vi "Calculate Q0 continous.vi"(8 "error in (no error)":errorcluster, 9 "dt":dbl=1e-06 format="%#_13g", 10 "Data":dbl[][](array[numeric]), 11 "Scope5761 in":refnum<class "Scope5782_six_channel.lvclass">) -> (0 "error out":errorcluster, 1 "Q0 error":bool, 2 "Data out":dbl[][](array[numeric]), 3 "Scope5761out":refnum<class "Scope5782_six_channel.lvclass">)   [LabVIEW 2025, in "Scope5782_six_channel.lvclass"]
uses:
  Scope5782_six_channel.lvclass
  Scope5782_six_channel.lvclass/Scope5782_six_channel.ctl
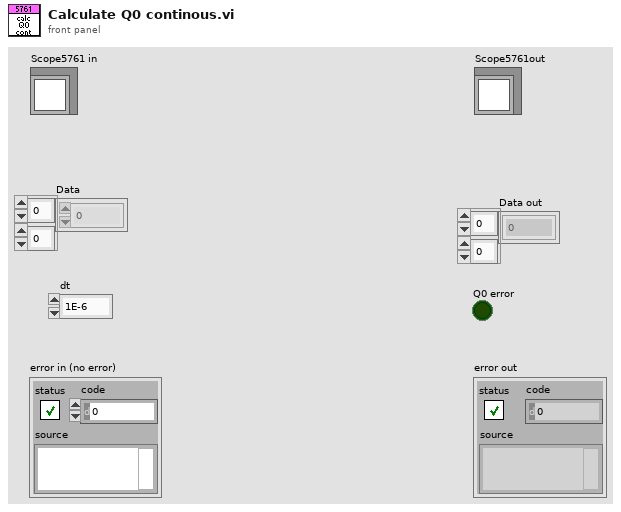
[diagram p1: front panel]
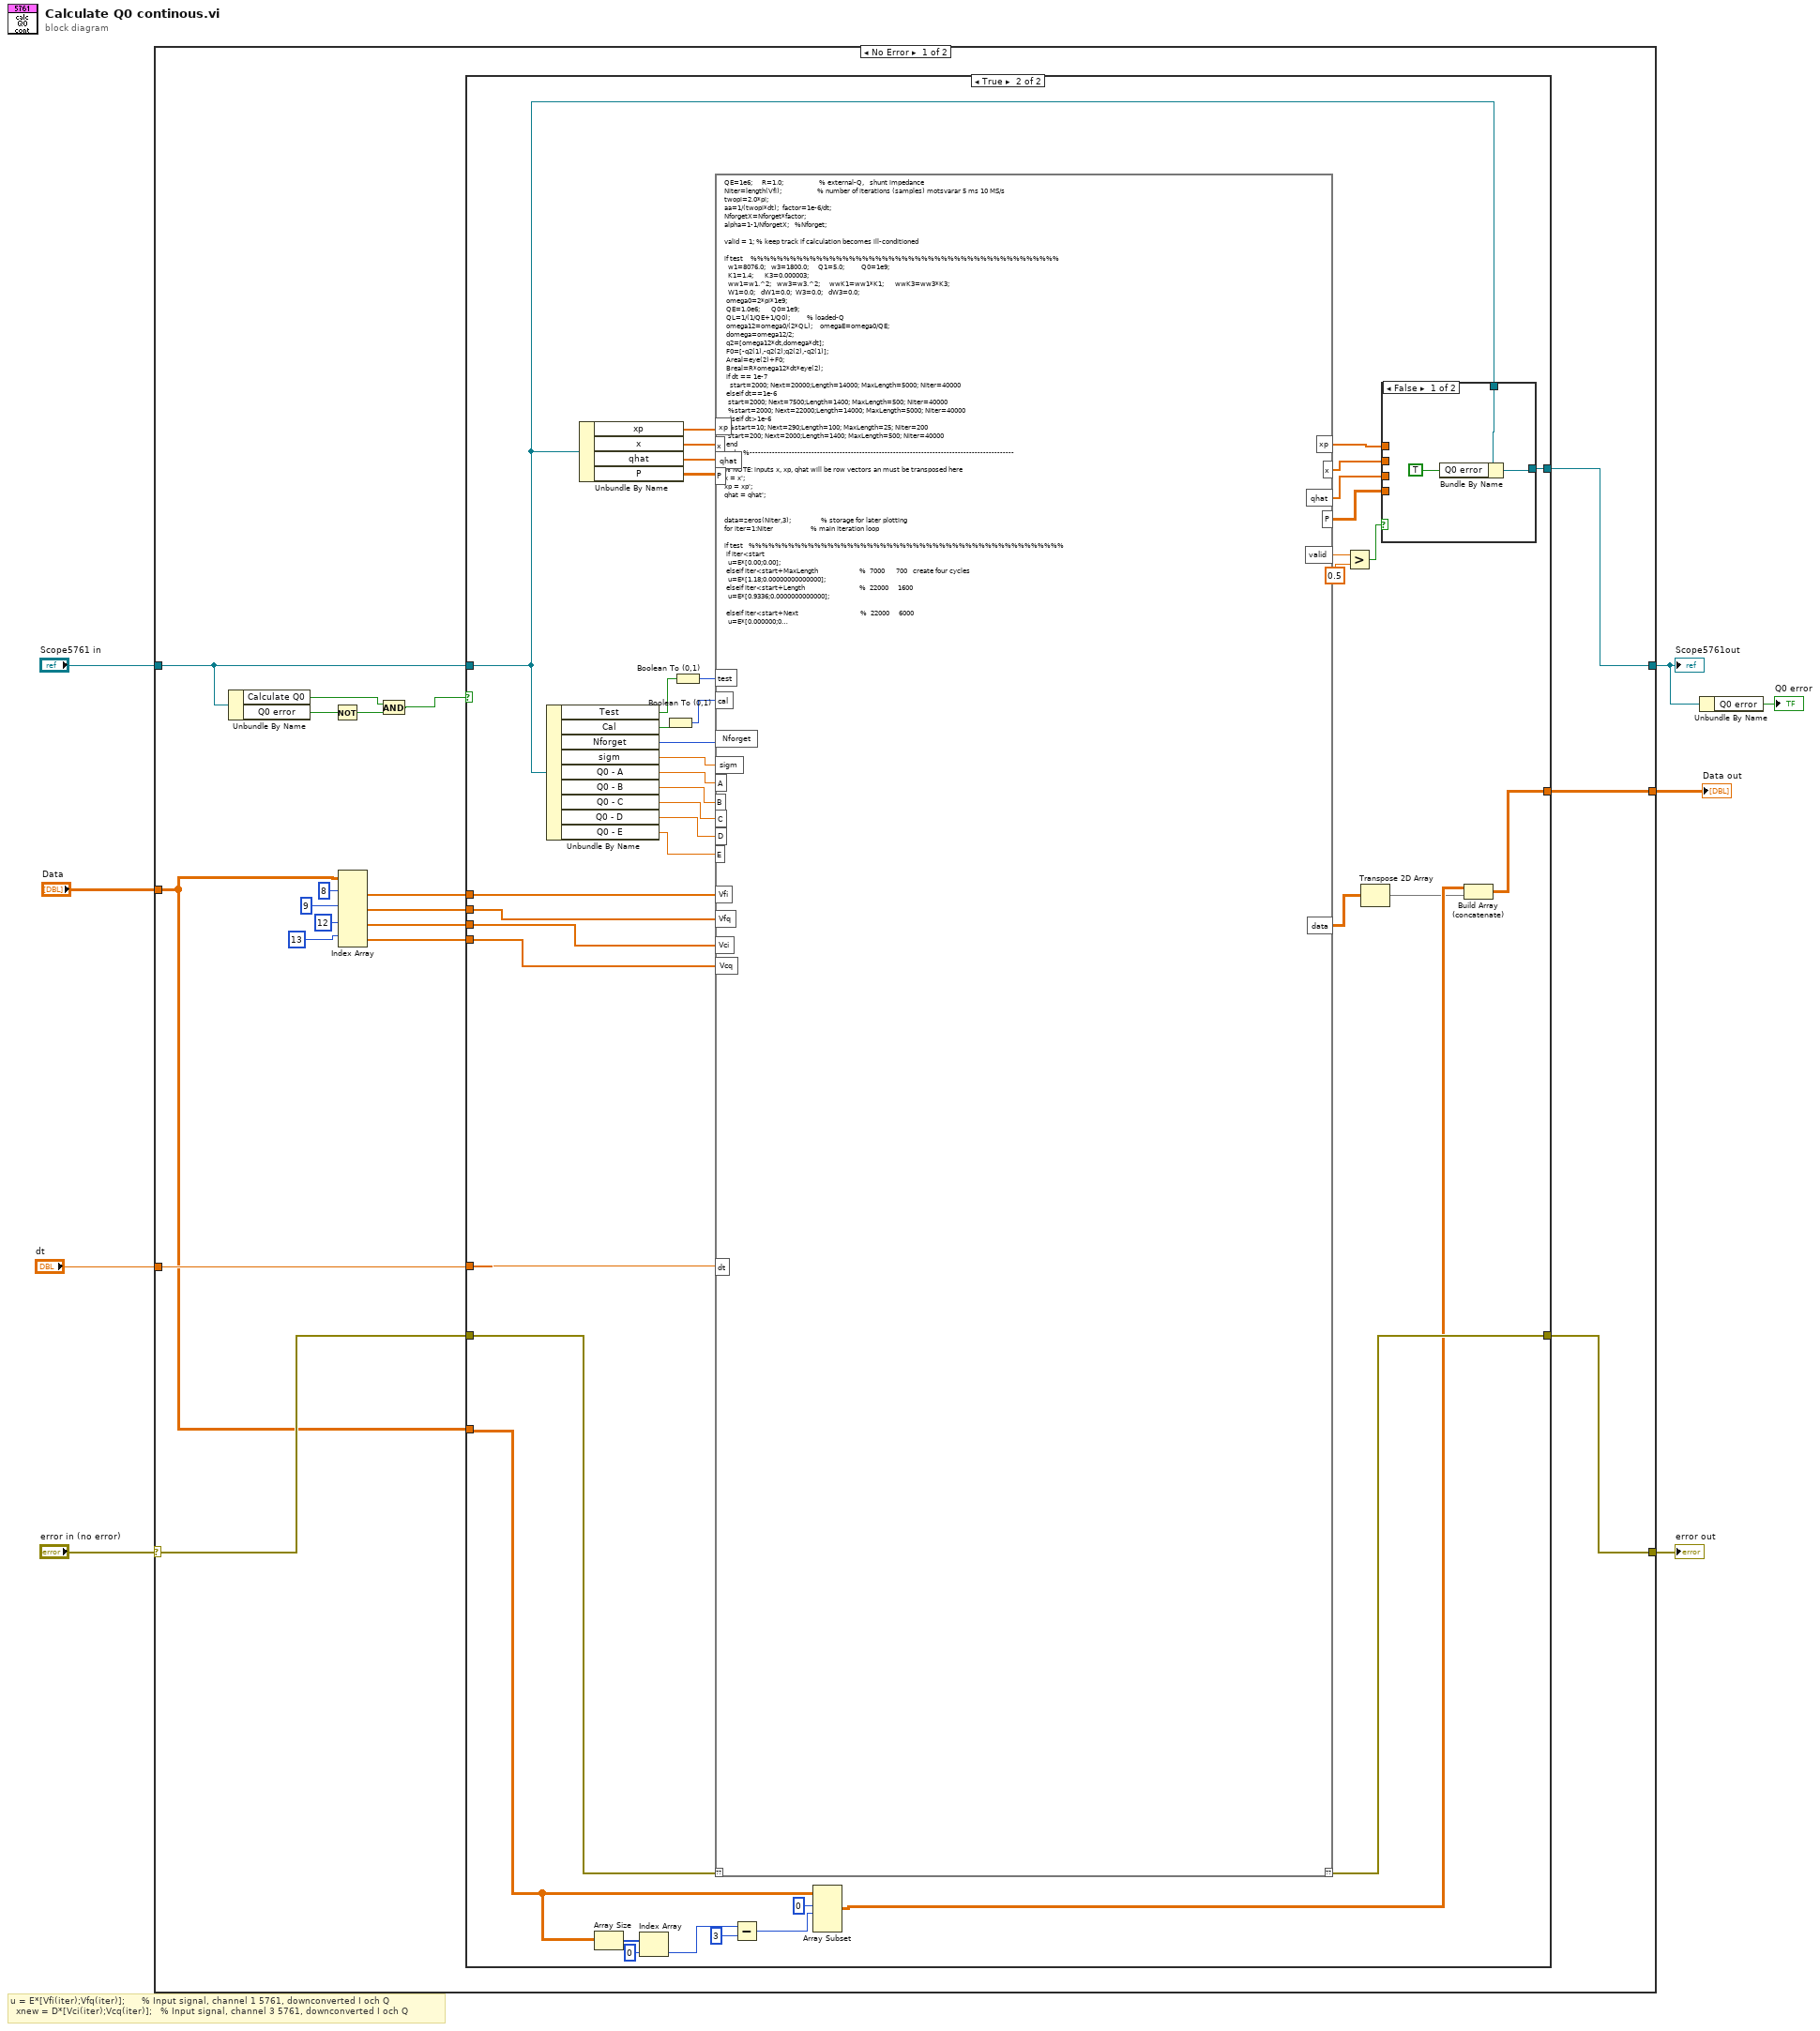
[diagram p0: block diagram]
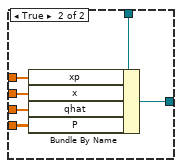
[diagram p3: hidden frame]
diagram:
  # "u = E*[Vfi(iter);Vfq(iter)];      % Input signal, channel 1 5761, downconverted I och Q \n  xnew = D*[Vci(iter);Vcq(iter)];   % Input signal, channel 3 5761, downconverted I och Q"
  n1 = case shown="No Error" "error in (no error)" {
    selector: "error in (no error)" -> [w21 w84]
    tunnel: [w20 w84] -> w7
    tunnel: [w15 w83] -> w2
    tunnel: "Scope5761 in" -> [w23 w83]
    tunnel: "Data" -> [w14 w82]
    tunnel: "dt" -> [w22 _]
    tunnel: [w13 w82] -> w3
    frame No Error {
      n2 = Unbundle By Name(w23) -> ("Calculate Q0"=w10:bool, "Q0 error"=w12:bool)
      n3 = Not(x=w12) -> (.not. x?=w11:bool)
      n4 = Index Array(array=w14, index (row) #1=8 ("index (row)"), index (row) #2=9 ("index (row)"), index (row) #3=12 ("index (row)"), index (row) #4=13 ("index (row)")) -> (element #1=w19:dbl[], element #2=w18:dbl[], element #3=w17:dbl[], element #4=w16:dbl[])  [unwired: 4 in]
      n5 = And(x=w10, y=w11) -> (x .and. y?=w9:bool)
      n6 = case shown="True" w9 {
        tunnel: w23 -> [w29 w39]
        tunnel: w22 -> [_ w65]
        tunnel: w21 -> [w30 w64]
        tunnel: [w30 w63] -> w20
        tunnel: w19 -> [_ w62]
        tunnel: w18 -> [_ w61]
        tunnel: w17 -> [_ w60]
        tunnel: w16 -> [_ w59]
        tunnel: [w29 w34] -> w15
        tunnel: w14 -> [w28 w48]
        tunnel: [w28 w50] -> w13
        frame False {
        }
        frame True {
          n7 = Unbundle By Name(w39) -> ("Test"=w47:bool, "Cal"=w45:bool, "Nforget"=w72:i32, "sigm"=w71:dbl, "Q0 - A"=w70:dbl, "Q0 - B"=w69:dbl, "Q0 - C"=w68:dbl, "Q0 - D"=w67:dbl, "Q0 - E"=w66:dbl)
          n8 = Unbundle By Name(w39) -> ("xp"=w43:dbl[], "x"=w42:dbl[], "qhat"=w41:dbl[], "P"=w40:dbl[][])
          n9 = Array Size(array=w48) -> (size(s)=w58:i32[])
          n10 = Index Array(array=w58, index=0) -> (element=w56:i32)
          n11 = Boolean To (0,1)(Boolean=w45) -> (0, 1=w44:i16)
          n12 = Boolean To (0,1)(Boolean=w47) -> (0, 1=w46:i16)
          n13 = script code="QE=1e6;     R=1.0;                   % external-Q,   shunt impedance\nNiter=length(Vfi);                   % number of iterations (samples) motsvarar 5 ms 10 MS/s\ntwopi=2.0*pi;\naa=1/(twopi*dt);  factor=1e-6/dt;\nNforgetX=Nforget*factor;\nalpha=1-1/NforgetX;   %Nforget; \n\nvalid = 1; % keep track if calculation becomes ill-conditioned\n\nif test    %%%%%%%%%%%%%%%%%%%%%%%%%%%%%%%%%%%%%%%%%%%%%%%\n  w1=8076.0;   w3=1800.0;     Q1=5.0;         Q0=1e9;            \n  K1=1.4;      K3=0.000003;   \n  ww1=w1.^2;   ww3=w3.^2;     wwK1=ww1*K1;      wwK3=ww3*K3;\n  W1=0.0;   dW1=0.0;  W3=0.0;   dW3=0.0;\n omega0=2*pi*1e9;\n QE=1.0e6;      Q0=1e9;                  \n QL=1/(1/QE+1/Q0);         % loaded-Q\n omega12=omega0/(2*QL);    omegaE=omega0/QE;         \n domega=omega12/2; \n q2=[omega12*dt,domega*dt];  \n F0=[-q2(1),-q2(2);q2(2),-q2(1)]; \n Areal=eye(2)+F0;       \n Breal=R*omega12*dt*eye(2);\n if dt == 1e-7\n   start=2000; Next=20000;Length=14000; MaxLength=5000; Niter=40000\n elseif dt==1e-6\n  start=2000; Next=7500;Length=1400; MaxLength=500; Niter=40000\n  %start=2000; Next=22000;Length=14000; MaxLength=5000; Niter=40000\n elseif dt>1e-6\n  %start=10; Next=290;Length=100; MaxLength=25; Niter=200\n  start=200; Next=2000;Length=1400; MaxLength=500; Niter=40000\n end\nend    %----------------------------------------------------------------------------------------------\n\n% NOTE: inputs x, xp, qhat will be row vectors an must be transposed here\nx = x';\nxp = xp';\nqhat = qhat';\n\n\ndata=zeros(Niter,3);                % storage for later plotting \nfor iter=1:Niter                    % main iteration loop\n\nif test   %%%%%%%%%%%%%%%%%%%%%%%%%%%%%%%%%%%%%%%%%%%%%%%%\n if iter<start\n  u=E*[0.00;0.00];\n elseif iter<start+MaxLength                      %  7000      700   create four cycles\n  u=E*[1.18;0.00000000000000];\n elseif iter<start+Length                             %  22000     1600\n  u=E*[0.9336;0.0000000000000];\n\n elseif iter<start+Next                                 %  22000     6000\n  u=E*[0.000000;0.0000000];\n elseif iter<start+Next+MaxLength          %  27000     6500\n  u=E*[1.180000;0.0000000];\n elseif iter<start+Next+Length                 %  36000     7400\n  u=E*[0.933600;0.0000000];\n\n elseif iter<start+2*Next                                 %  42000     6000\n  u=E*[0.000000;0.0000000];\n elseif iter<start+2*Next+MaxLength          %  65000     6500\n  u=E*[1.180000;0.0000000];\n elseif iter<start+2*Next+Length                 %  80000     7400\n  u=E*[0.933600;0.0000000];\n\nelseif iter<start+3*Next                                 %  60000     6000\n  u=E*[0.000000;0.0000000];\nelseif iter<start+3*Next+MaxLength          %  65000     6500\n  u=E*[1.180000;0.0000000];\nelseif iter<start+3*Next+Length                 %  80000     7400\n  u=E*[0.933600;0.0000000];\n\nelse     %if iter<start+3*Next                    %  118000  11800\n  u=E*[0.000000;0.0000000];\nend\n  %.........................................cavity dynamics\n  xpnew=Areal*xp+Breal*u+0.000001*randn(size(x)); % eq. 2, xp=V\n  xnew=xpnew+sigm*0.001*randn(size(x));        % xnew=V', add measurement noise\n  %...................................system identification\n  u=u*QE/(2*QL);  \n  y=D*(xnew-x); \nend    %----------------------------------------------------------------------------------------------\n\n if ~test   %%%%%%%%%%%%%%%%%%%%%%%%%%%%%%%%%%%%%%%%%%%%%\n  u = E*[Vfi(iter);Vfq(iter)];      % Input signal, channel 1 5761, downconverted I och Q \n  xnew = D*[Vci(iter);Vcq(iter)];   % Input signal, channel 3 5761, downconverted I och Q \n\n  if iter < 2\n    y = aa*(xnew-x);\n  else\n    x = D*[Vci(iter-1);Vcq(iter-1)];  % Input signal, channel 3\n    y = aa*(xnew-x) + sigm*randn(size(x));\n  end\n end  %-----------------------------------------------------------------------------------------------\n\n  %...........Matrix Math (G=[3,2], G'=[2,3], P=[3,3]).....................\n  G=[-0.5*x(1)+u(1)*R,-x(2),-0.5*x(1);-0.5*x(2)+u(2)*R,x(1),-0.5*x(2)];\n  tmp2=eye(3)-P*G'*inv(alpha*eye(2)+G*P*G')*G;    \n  Pnew=tmp2*P/alpha; \n  qhat=tmp2*(qhat+P*G'*y/alpha);\n\n if test    %%%%%%%%%%%%%%%%%%%%%%%%%%%%%%%%%%%%%%%%%%%%%%%\n  vv2=xnew'*xnew;\n  sqV=2.01*(1e1)*vv2; % to mechanical part\n  W1new  = W1 + dW1*dt;\n  dW1new = dW1 + (-ww1*W1-(w1/Q1)*dW1-wwK1*sqV)*dt; \n  W3new  = W3 + dW3*dt;\n  dW3new = dW3 + (-ww3*W3-(w3/Q1)*dW3-wwK3*sqV)*dt;  \n  dwdt = (W1+W3)*dt;\n  Areal(1,2)= -dwdt; % to electrical part in next iteration\n  Areal(2,1)= dwdt;  % to electrical part in next iteration\n  W1=W1new;  dW1=dW1new;  W3=W3new;  dW3=dW3new;\n  xp=xpnew;                                                    \n end  %-----------------------------------------------------------------------------------------------\n\n  x=xnew;  \n  P=Pnew;\n\n  %...........Matrix Math end..............................................\n  %................................save for later plotting \n  data(iter,1)= u(1); %qhat(1)*A*factor;           % Output signal, fE (omegaE/twopi)   \n  data(iter,2)=qhat(2)*B*factor;           % Output signal, d_f (detuning/twopi)  \n  data(iter,3)=qhat(3)*C*factor;           % Output signal, fQ0 (omega00/twopi) \n  \n  valid = valid & all(isfinite(data(iter, :)));\n  if(~valid)\n      break;\n  end\nend\n\nvalid = double(valid);\n\n% NOTE: transpose  x, xp, qhat cak to rows\nx = x';\nxp = xp';\nqhat = qhat';"("??"=w64, "Nforget"=w72, "sigm"=w71, "dt"=w65, "A"=w70, "B"=w69, "C"=w68, "D"=w67, "E"=w66, "Vfi"=w62, "Vfq"=w61, "Vci"=w60, "Vcq"=w59, "test"=w46, "cal"=w44, "xp"=w43, "x"=w42, "qhat"=w41, "P"=w40) -> ("??"=w63:errorcluster, "data"=w51:dbl[][], "xp"=w38:dbl[], "x"=w37:dbl[], "qhat"=w36:dbl[], "P"=w35:dbl[][], "valid"=w33:dbl)
          n14 = Subtract(x=w56, y=3) -> (x-y=w54:i32)
          n15 = Array Subset(array=w48, index (row)=0 ("index"), length (row)=w54) -> (w52:dbl[][])  [unwired: 2 in]
          n16 = Greater?(x=w33, y=0.5) -> (0:w31:bool)
          n17 = Transpose 2D Array(2D array=w51) -> (transposed array=w49:dbl[][])
          n18 = case shown="False" w31 {
            tunnel: w39 -> [w74 w81]
            tunnel: w38 -> [_ w80]
            tunnel: w37 -> [_ w79]
            tunnel: w36 -> [_ w78]
            tunnel: w35 -> [_ w77]
            tunnel: [w75 w76] -> w34
            frame False {
              n19 = Bundle By Name(cluster=w74, "Q0 error"=TRUE) -> (w75:refnum<class "Scope5782_six_channel.lvclass">)
            }
            frame True {
              n20 = Bundle By Name(cluster=w81, "xp"=w80, "x"=w79, "qhat"=w78, "P"=w77) -> (w76:refnum<class "Scope5782_six_channel.lvclass">)
            }
          }
          n21 = Build Array (concatenate)(w52, w49) -> (w50:dbl[][])
        }
      }
    }
    frame Error {
    }
  }
  "error out" <- w7
  "Scope5761out" <- w2
  "Data out" <- w3
  n22 = Unbundle By Name(w2) -> ("Q0 error"=→"Q0 error":bool)
